vi "trajectoryManager.vi"(0 "Game in":refnum<class "Game.lvclass">, 1 "v_tang_curve":dbl format="%#_13g", 2 "v_ang_curve":dbl format="%#_13g", 5 "Robot":refnum<class "Robot.lvclass">, 9 "Dest_array":T2(array[cluster]), 11 "error in (no error)":errorcluster, 12 "firstCall":bool=TRUE, 14 "traj_state":T1=enum."circle") -> (3 "next_dest":dbl[](array[numeric]) format="%#_13g", 4 "Game out":refnum<class "Game.lvclass">, 6 "Dest":dbl[](array[numeric]) format="%#_13g", 8 "v_desired":dbl format="%#_13g", 10 "traj_state out":T1=enum."circle", 13 "last_dest":bool, 15 "error out":errorcluster)   [LabVIEW 2020, in "Game.lvclass"]
uses:
  Game.lvclass
  Robot_class/Robot.lvclass
  C:/RoboIME/SSL_AI/Object_class/Object.lvclass
  Controls/trajectoryState.ctl
  Object_class/Object.lvclass/Object.ctl
  Object_class/Read x.vi
  Object_class/Read y.vi
  <vilib>/Analysis/_algsub.llb/Real Vector Norm.vi
  Utilities_class/Utilities.lvclass
  <vilib>/Analysis/NI_AALPro.lvlib
panel:
  out "angleBetweenVectors":dbl
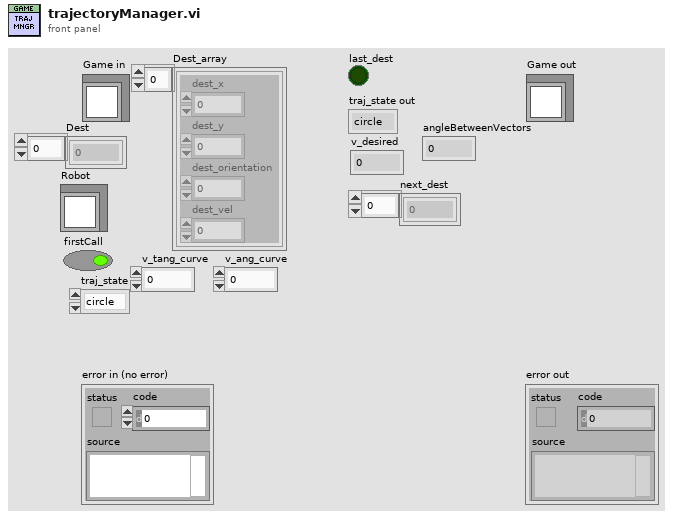
[diagram p1: front panel]
types:
  T1 = typedef "trajectoryState.ctl" = enum16{"replace", "circle", "line"}
  T2 = cluster{"dest_x":dbl, "dest_y":dbl, "dest_orientation":dbl, "dest_vel":dbl}[]
  T3 = cluster{"dest_x":dbl, "dest_y":dbl, "dest_orientation":dbl, "dest_vel":dbl}
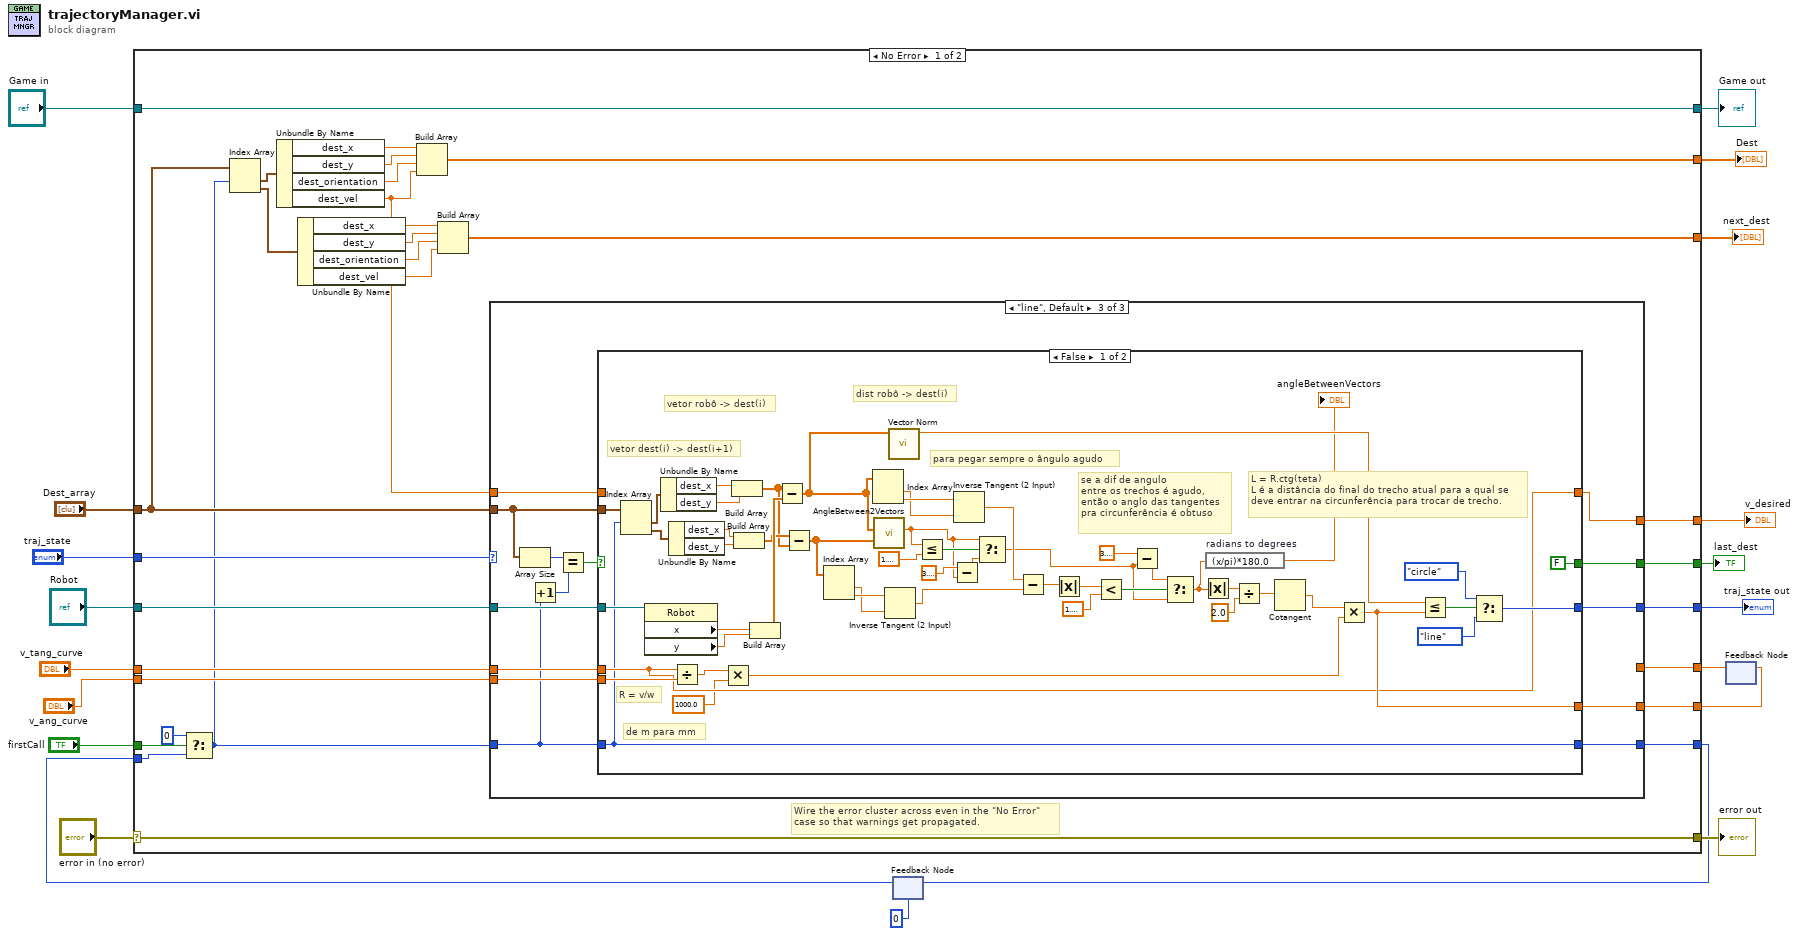
[diagram p0: block diagram]
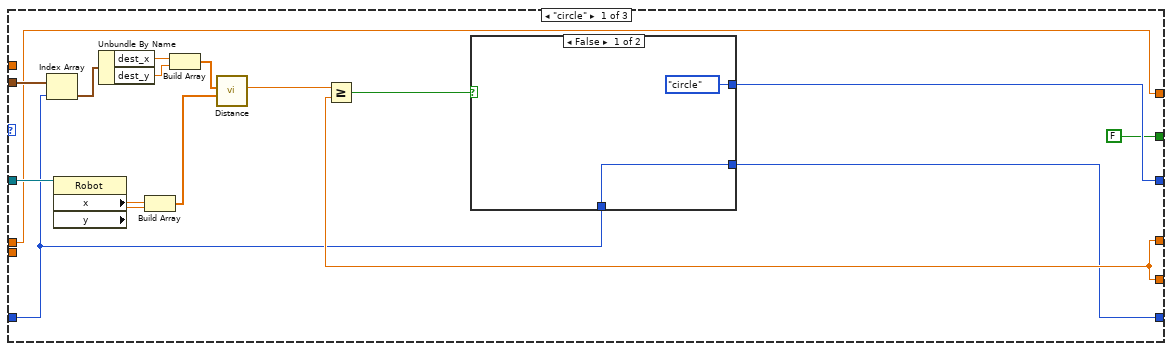
[diagram p2: hidden frame]
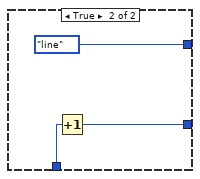
[diagram p3: hidden frame]
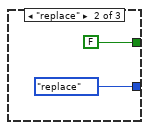
[diagram p4: hidden frame]
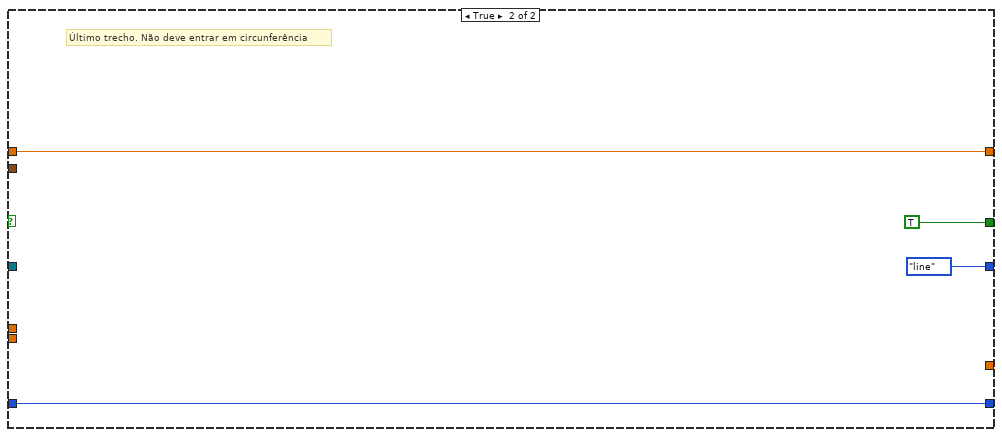
[diagram p5: hidden frame]
diagram:
  n1 = feedback #1(0 ("index")) -> (w12:i32)
  n2 = feedback #2() -> (w4:dbl)  [unwired: 1 in]
  n3 = case shown="No Error" "error in (no error)" {
    selector: "error in (no error)" -> [w48 w145]
    tunnel: [w48 w145] -> w19
    tunnel: [w49 w144] -> w17
    tunnel: "Game in" -> [w49 w144]
    tunnel: "Dest_array" -> [w38 _]
    tunnel: "Robot" -> [w43 _]
    tunnel: "firstCall" -> [w46 _]
    tunnel: w12 -> [w44 _]
    tunnel: "traj_state" -> [w47 _]
    tunnel: "v_tang_curve" -> [w42 _]
    tunnel: "v_ang_curve" -> [w41 _]
    tunnel: [w40 _] -> w8
    tunnel: [w39 _] -> w7
    tunnel: [w32 _] -> w6
    tunnel: [w31 _] -> w5
    tunnel: w4 -> [w30 _]
    tunnel: [w28 _] -> w3
    tunnel: [w27 _] -> w2
    tunnel: [w21 _] -> w1
    frame No Error {
      # "Wire the error cluster across even in the \"No Error\"\ncase so that warnings get propagated."
      n4 = Select(t=0 ("index"), s=w46, f=w44) -> (s? t:f=w37:i32)
      n5 = Index Array(array=w38, index #1=w37) -> (element #1=w36:T3, element #2=w24:T3)  [unwired: 1 in]
      n6 = Unbundle By Name(w36) -> ("dest_x"=w35:dbl, "dest_y"=w34:dbl, "dest_orientation"=w33:dbl, "dest_vel"=w29:dbl)
      n7 = Unbundle By Name(w24) -> ("dest_x"=w26:dbl, "dest_y"=w25:dbl, "dest_orientation"=w23:dbl, "dest_vel"=w22:dbl)
      n8 = Build Array(w35, w34, w33, w29) -> (w32:dbl[])
      n9 = Build Array(w26, w25, w23, w22) -> (w21:dbl[])
      n10 = case shown="\"line\", Default" w47 {
        tunnel: w38 -> [w65 _ w83]
        tunnel: w37 -> [w53 _ w80]
        tunnel: w43 -> [w60 _ w87]
        tunnel: w42 -> [w51 _ w86]
        tunnel: w41 -> [_ _ w85]
        tunnel: [w52 _ w78] -> w40
        tunnel: [w54 trajectoryState."replace" ("traj_state") w84] -> w39
        tunnel: [w56 _ w77] -> w31
        tunnel: w30 -> [w56 _ _]
        tunnel: w29 -> [_ _ w76]
        tunnel: [w51 _ w75] -> w28
        tunnel: [FALSE FALSE w74] -> w27
        frame "circle" {
          n11 = Index Array(array=w65, index=w53) -> (element=w64:T3)
          n12 = property class="Robot"(reference=w60) -> ("x"=w61:dbl, "y"=w62:dbl)  [unwired: 1 in, 2 out]
          n13 = Unbundle By Name(w64) -> ("dest_x"=w66:dbl, "dest_y"=w63:dbl)
          n14 = Build Array(w61, w62) -> (w58:dbl[])
          n15 = Build Array(w66, w63) -> (w59:dbl[])
          n16 = call "Distance.vi"("P1"=w58, "P2"=w59) -> ("Distance"=w57:dbl)  [unwired: 7 in, 2 out]
          n17 = Greater Or Equal?(x=w57, y=w56) -> (x >= y?=w55:bool)
          n18 = case shown="False" w55 {
            tunnel: [trajectoryState."circle" ("traj_state") trajectoryState."line" ("traj_state")] -> w54
            tunnel: w53 -> [w68 w70]
            tunnel: [w68 w69] -> w52
            frame False {
            }
            frame True {
              n19 = Increment(x=w70) -> (x+1=w69:i32)
            }
          }
        }
        frame "replace" {
        }
        frame "line", Default {
          n20 = Array Size(array=w83) -> (size(s)=w82:i32)
          n21 = Increment(x=w80) -> (x+1=w81:i32)
          n22 = Equal?(x=w82, y=w81) -> (x = y?=w79:bool)
          n23 = case shown="False" w79 {
            tunnel: w83 -> [w139 _]
            tunnel: w87 -> [w135 _]
            tunnel: w86 -> [w103 _]
            tunnel: w85 -> [w115 _]
            tunnel: w80 -> [w88 w142]
            tunnel: [w105 trajectoryState."line" ("traj_state")] -> w84
            tunnel: [w88 w142] -> w78
            tunnel: [w104 _] -> w77
            tunnel: [w103 w141] -> w75
            tunnel: w76 -> [_ w141]
            tunnel: [FALSE TRUE] -> w74
            frame False {
              # "de m para mm"
              # "dist robô -> dest(i)"
              # "vetor dest(i) -> dest(i+1)"
              # "vetor robô -> dest(i)"
              # "L = R.ctg(teta)\nL é a distância do final do trecho atual para a qual se\ndeve entrar na circunferência para trocar de trecho."
              # "se a dif de angulo\nentre os trechos é agudo,\nentão o anglo das tangentes\npra circunferência é obtuso"
              # "para pegar sempre o ângulo agudo"
              # "R = v/w"
              n24 = Index Array(array=w139, index #1=w88) -> (element #1=w138:T3, element #2=w133:T3)  [unwired: 1 in]
              n25 = property class="Robot"(reference=w135) -> ("x"=w129:dbl, "y"=w130:dbl)  [unwired: 1 in, 2 out]
              n26 = Unbundle By Name(w138) -> ("dest_x"=w137:dbl, "dest_y"=w136:dbl)
              n27 = Unbundle By Name(w133) -> ("dest_x"=w132:dbl, "dest_y"=w131:dbl)
              n28 = Divide(x=w103, y=w115) -> (x/y=w98:dbl)
              n29 = Multiply(x=w98, y=1000.0) -> (x*y=w97:dbl)
              n30 = Build Array(w137, w136) -> (w111:dbl[])
              n31 = Build Array(w132, w131) -> (w112:dbl[])
              n32 = Build Array(w129, w130) -> (w134:dbl[])
              n33 = Subtract(x=w111, y=w134) -> (x-y=w110:dbl[])
              n34 = Subtract(x=w112, y=w111) -> (x-y=w126:dbl[])
              n35 = Index Array(array=w126) -> (element #1=w124:dbl, element #2=w125:dbl)  [unwired: 2 in]
              n36 = Index Array(array=w110) -> (element #1=w127:dbl, element #2=w128:dbl)  [unwired: 2 in]
              n37 = call "AngleBetween2Vectors.vi"("Array 1"=w126, "Array 2"=w110) -> ("angleInRadians(default)"=w90:dbl)  [unwired: 6 in, 3 out]
              n38 = Inverse Tangent (2 Input)(1:w124, 2:w125) -> (0:w122:dbl)
              n39 = call-poly <vilib>:"Vector Norm.vi"("Input Vector"=w110) -> ("norm"=w109:dbl)  [unwired: 9 in, 1 out]
              n40 = Less Or Equal?(x=w90, y=1.5707963267948966) -> (x <= y?=w93:bool)
              n41 = Subtract(x=3.141592653589793, y=w90) -> (x-y=w91:dbl)
              n42 = Inverse Tangent (2 Input)(1:w127, 2:w128) -> (0:w123:dbl)
              n43 = Select(t=w90, s=w93, f=w91) -> (s? t:f=w89:dbl)
              n44 = Subtract(x=w123, y=w122) -> (x-y=w121:dbl)
              n45 = Absolute Value(x=w121) -> (abs(x)=w120:dbl)
              n46 = Less?(x=w120, y=1.5707963267948966) -> (x < y?=w118:bool)
              n47 = Subtract(x=3.141592653589793, y=w89) -> (x-y=w116:dbl)
              n48 = Select(t=w116, s=w118, f=w89) -> (s? t:f=w101:dbl)
              n49 = Absolute Value(x=w101) -> (abs(x)=w100:dbl)
              n50 = expression code="(x/pi)*180.0" "radians to degrees"(w101) -> (→"angleBetweenVectors":dbl)
              n51 = Divide(x=w100, y=2.0) -> (x/y=w114:dbl)
              n52 = Cotangent(1:w114) -> (0:w113:dbl)
              n53 = Multiply(x=w113, y=w97) -> (x*y=w104:dbl)
              n54 = Less Or Equal?(x=w109, y=w104) -> (x <= y?=w108:bool)
              n55 = Select(t=trajectoryState."circle" ("traj_state"), s=w108, f=trajectoryState."line" ("traj_state")) -> (s? t:f=w105:T1)
            }
            frame True {
              # "Último trecho. Não deve entrar em circunferência"
            }
          }
        }
      }
    }
    frame Error {
    }
  }
  "error out" <- w19
  "Game out" <- w17
  "Dest" <- w6
  "traj_state out" <- w7
  "v_desired" <- w3
  "last_dest" <- w2
  "next_dest" <- w1
  n56 = feedback-in #1(w8) -> ()
  n57 = feedback-in #2(w5) -> ()
